vi "Defer Panel Updates (Close).vi"(8 "error in (no error)":errorcluster, 10 "Panel refs":refnum<vi>[](array[refnum]), 11 "Registry Control Reference Accessor in":refnum<class "Registry Ctrl Ref Accessor.lvclass">) -> (0 "error out":errorcluster, 3 "Registry Control Reference Accessor out":refnum<class "Registry Ctrl Ref Accessor.lvclass">)   [LabVIEW 2013, in "Registry Ctrl Ref Accessor.lvclass"]
doc: "Copyright 2018, Carya Automatisering, Wiebe Walstra."
uses:
  Registry Ctrl Ref Accessor.lvclass
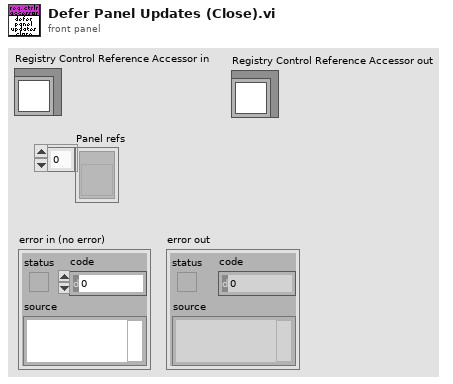
[diagram p1: front panel]
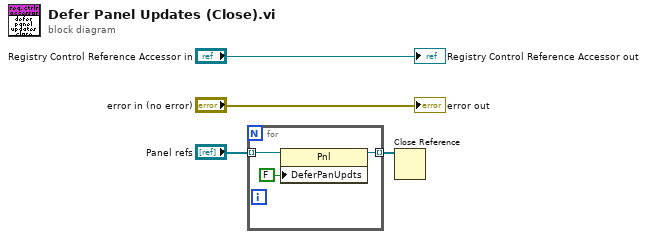
[diagram p0: block diagram]
diagram:
  n1 = for {
    tunnel: "Panel refs" -> [w6] mode=indexing
    tunnel: [w5] -> w1 mode=indexing
    n2 = property class="Pnl"(reference=w6, "DeferPanUpdts"=FALSE ("Defer Panel Updates")) -> (reference out=w5:refnum<vi>)  [unwired: 1 in, 1 out]
  }
  n3 = Close Reference(reference=w1) -> ()  [unwired: 1 in, 1 out]
  "error out" <- "error in (no error)"
  "Registry Control Reference Accessor out" <- "Registry Control Reference Accessor in"
